vi "AssetMgrGetMappedDataGroupAssetsRequest_Create.vi"(7 "Header":T2, 8 "error in (no error)":errorcluster, 9 "AssetMgrGetMappedDataGroupAssetsRequest":T1, 11 "ReplyTo":string) -> (0 "error out":errorcluster, 3 "Message":T4)   [LabVIEW 2017]
uses:
  <vilib>/addons/InsightCM/MessageBus/Base/controls/Message.ctl
  <vilib>/addons/InsightCM/MessageBus/Base/controls/MessageHeader.ctl
  <vilib>/addons/InsightCM/MessageBus/Base/controls/KeyValuePair.ctl
  <vilib>/addons/InsightCM/MessageBus/MessageLibrary/AssetManager/controls/AssetMgrGetMappedDataGroupAssetsRequestBody.ctl
  <vilib>/addons/InsightCM/MessageBus/Base/controls/MessageClassType.ctl
  <vilib>/addons/InsightCM/Utilities/PropertyHelpers/PropertyHelpers.lvlib
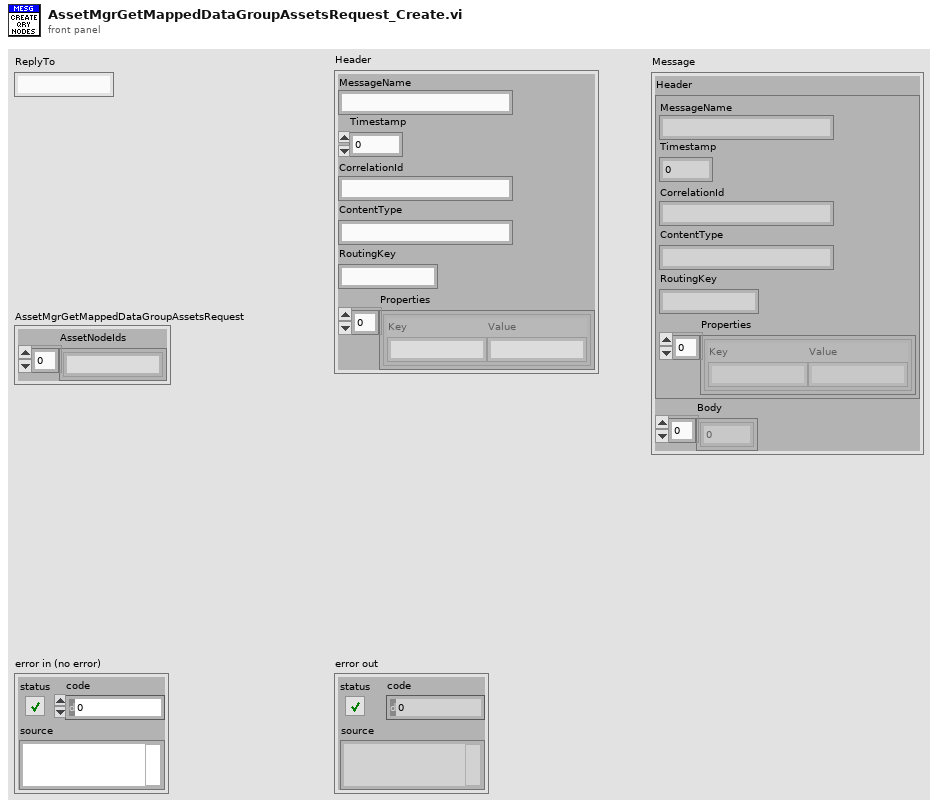
[diagram p1: front panel]
types:
  T1 = typedef "AssetMgrGetMappedDataGroupAssetsRequestBody.ctl" = cluster{"AssetNodeIds":string[]}
  T2 = typedef "MessageHeader.ctl" = cluster{"MessageName":string, "Timestamp":i64, "CorrelationId":string, "ContentType":string, "RoutingKey":string, "Properties":T3[]}
  T3 = typedef "KeyValuePair.ctl" = cluster{"Key":string, "Value":string}
  T4 = typedef "Message.ctl" = cluster{"Header":T2, "Body":u8[]}
  T5 = typedef "MessageClassType.ctl" = enum16{"Request", "Response", "Broadcast", "RoutedMessage"}
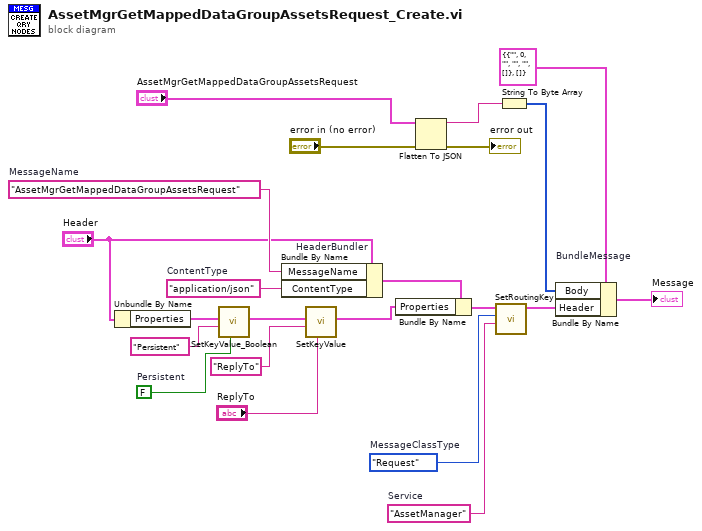
[diagram p0: block diagram]
diagram:
  w18 = MessageClassType."Request"  # MessageClassType
  w3 = "AssetManager"  # Service
  w13 = FALSE  # Persistent
  w19 = "AssetMgrGetMappedDataGroupAssetsRequest"  # MessageName
  w16 = "application/json"  # ContentType
  n1 = Unbundle By Name("Header") -> ("Properties"=w15:T3[])
  n2 = call <vilib>:"SetKeyValue_Boolean.vi"("value"=w13, "key"="Persistent" ("Key"), "key value pairs"=w15) -> ("key value pairs out"=w11:T3[])  [unwired: 8 in]
  n3 = Bundle By Name "HeaderBundler"(cluster="Header", "MessageName"=w19, "ContentType"=w16) -> (w9:T2)
  n4 = call <vilib>:"SetKeyValue.vi"("value"="ReplyTo", "key"="ReplyTo" ("Key"), "key value pairs"=w11) -> ("key value pairs out"=w8:T3[])  [unwired: 8 in]
  n5 = Bundle By Name(cluster=w9, "Properties"=w8) -> (w10:T2)
  n6 = Flatten To JSON(anything="AssetMgrGetMappedDataGroupAssetsRequest", error in (no error)="error in (no error)") -> (JSON string=w2:string, 11:→"error out":errorcluster)  [unwired: 1 in]
  n7 = call <vilib>:"SetRoutingKey.vi"("SendTo"=w3, "MessageClassType"=w18, "Message Header in"=w10) -> ("Message Header out"=w12:T2)  [unwired: 8 in]
  n8 = String To Byte Array(string=w2) -> (unsigned byte array=w21:u8[])
  n9 = Bundle By Name "BundleMessage"(cluster=T4 {"Header"={"MessageName"="", "Timestamp"=0, "CorrelationId"="", "ContentType"="", "RoutingKey"="", "Properties"=[]}, "Body"=[]} ("Message"), "Body"=w21, "Header"=w12) -> (→"Message":T4)
